vi "basic_serial_write_and_read.vi"(0 "VISA resource name":refnum<visa-resource-name>="COM1", 1 "baud rate":u32=9600, 2 "data bits":u16=8 min=5 max=8 step=1, 3 "parity":u16(ring) items=["None", "Odd", "Even", "Mark", "Space"], 4 "stop bits":u16(ring)=10 items=["1.0"=10, "1.5"=15, "2.0"=20], 7 "flow control":u16(ring) items=["None"=0, "XON/XOFF"=1, "RTS/CTS"=2, "DTR/DSR"=4], 10 "bytes to read":u32=5) -> (9 "read string":string)   [LabVIEW 2017]
doc: "The Basic Serial Read and Write example performs a Serial Port Read, a Serial Port Write, or a combination of these actions. The user selects the actions (read or write) on the front panel. If both are selected, the VI will write the data first, read data, and then close the VISA session that is opened to the port. This VI will wait until the specified number of bytes is received at the port. Only the number of bytes specified will be read.\n\nINSTRUCTIONS:\n1) Select the serial resource and configuration parameters (baud rate, data bits, parity, stop bits, flow control).\n2) Select the operations to be performed. \n3) Connect the serial port to your device. If no device is available, perform a loopback test by doing one of the following. Short pins 2 and 3 on a RS-232 cable or short pin 4 to pin 8 and pin 5 to pin 9 on a RS-485/422 cable. \n4) Run the VI to see the data read. (The \"read string\" will match the \"string to write\" if a loopback test was performed.)\n\nNote: The parameters set for the serial port must match the parameters of the connected instrument or device. In this example, the bytes to read parameter specifies the number of bytes that the serial port reads. If there were more bytes at the port than the number specified in bytes to read, those bytes would not be read. Also, if you specify to read more bytes than the number of bytes actually read, you might receive a timeout error message.\n\nOn the block diagram, the Configure Serial Port VI sets the configuration parameters. The front panel displays the controls used to configure the basic parameters, such as baud rate, data bits, and parity. Constants configure the other parameters the user probably does not need set. After the VISA Configure Serial Port VI opens the VISA session and configures the port, the VI passes the VISA resource name to other VIs that perform operations on that VISA resource. The VISA Write function sends a command to the serial device and the VISA Read function returns data based on the command. The VISA Close function then closes the reference to the serial device. It is important to close the reference; otherwise communication through with that port through protocols other than VISA might not be possible."
uses:
  <vilib>/Instr/_visa.llb/VISA Configure Serial Port (Instr).vi
panel:
  out "x-y":dbl
  out "S2":dbl
  out "S1":dbl
  out "S2":dbl
  out "S1":dbl
  out "output 2":dbl
  out "output 1":dbl
  in  "stop 2":bool
  out "concatenated string":string
  in  "stop":bool
  # "Select the serial resource and the operations (Read, Write, or both) to be performed.  If both are selected, the VI will write the data first, read data and then close the VISA session that is opened to the port.  This VI will wait until the specified number of bytes is received at the port. Only the number of bytes specified will be read."
  # "For additional information select File >> VI Properties >> Documentation"
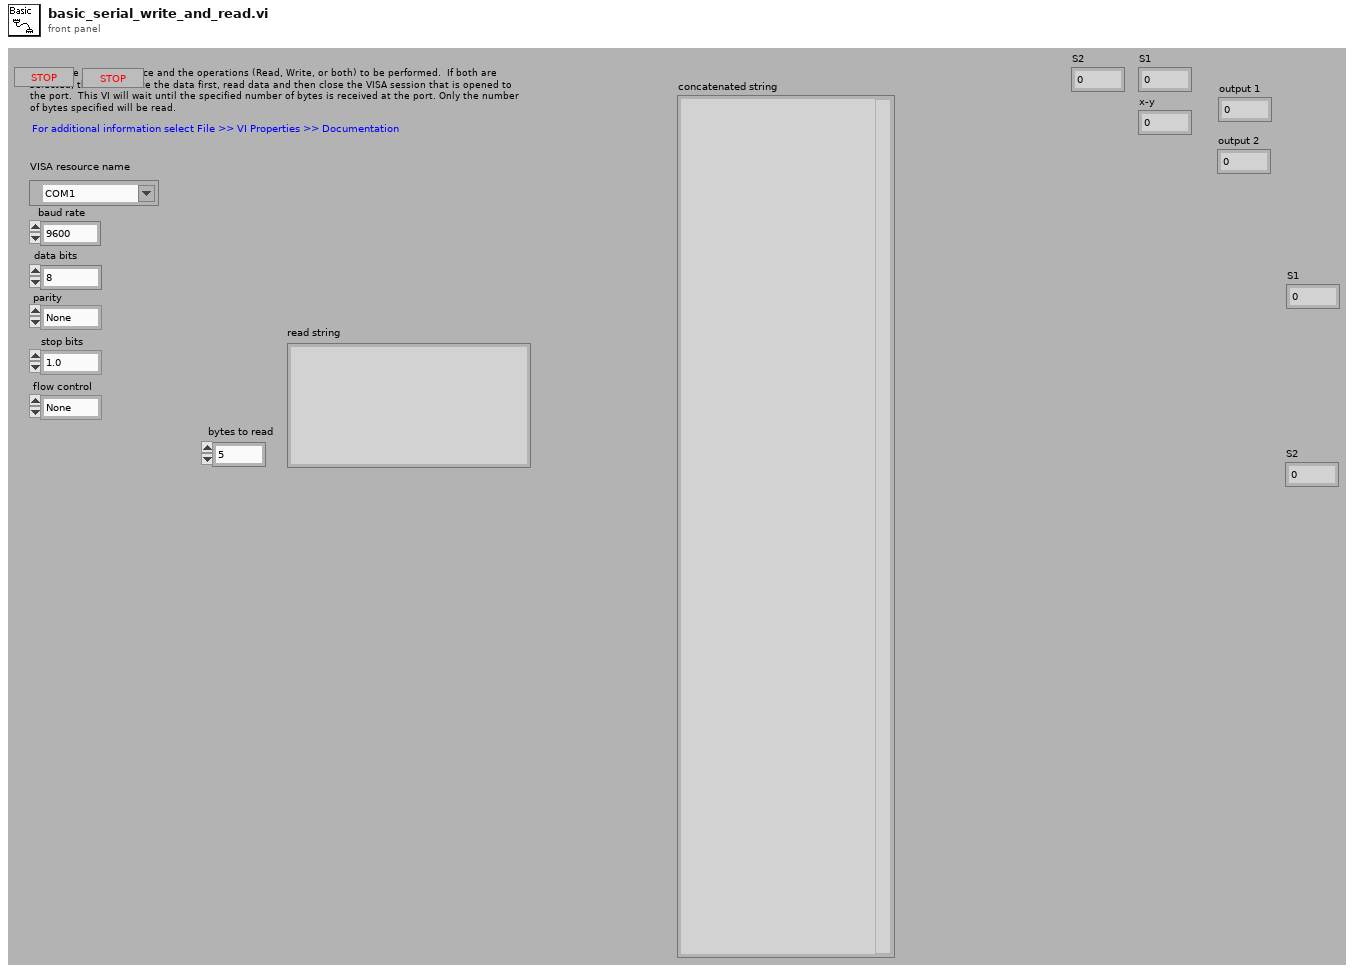
[diagram p1: front panel]
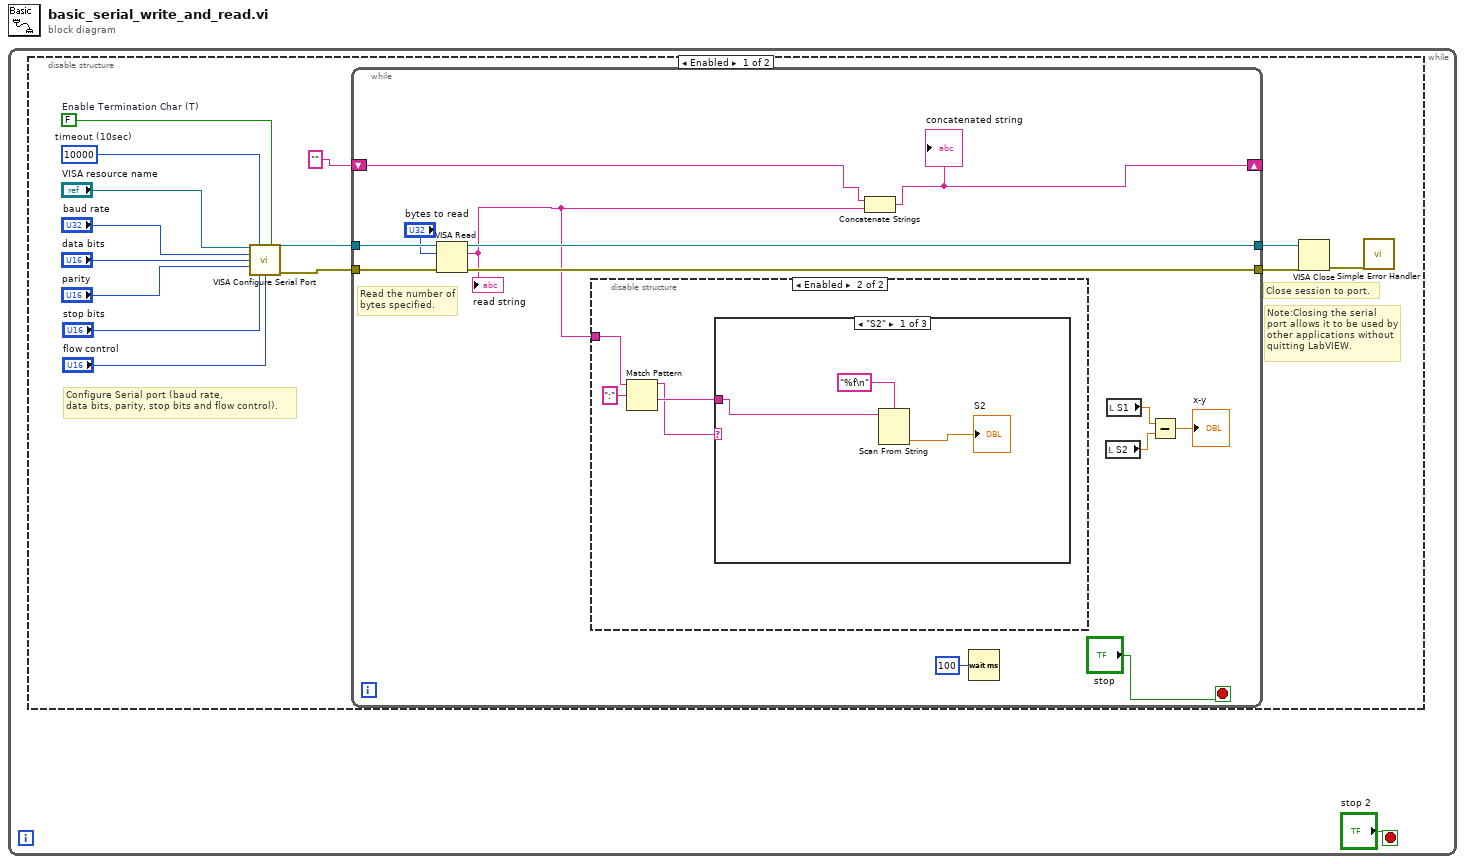
[diagram p0: block diagram]
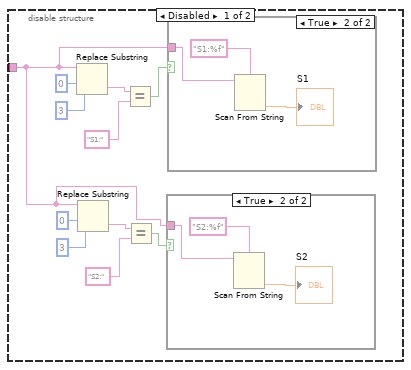
[diagram p2: hidden frame]
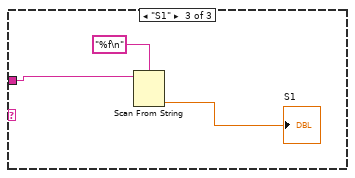
[diagram p6: hidden frame]
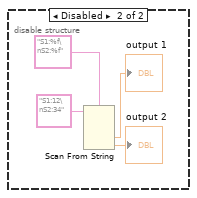
[diagram p7: hidden frame]
diagram:
  n1 = while {
    stop <- "stop 2" stop-if-true
    n2 = disable-structure shown="Enabled" {
      frame Enabled {
        w8 = FALSE  # Enable Termination Char (T)
        w9 = u32 10000  # timeout (10sec)
        # "Note:Closing the serial port allows it to be used by other applications without\nquitting LabVIEW."
        # "Close session to port."
        # "Configure Serial port (baud rate,\ndata bits, parity, stop bits and flow control)."
        n3 = call-poly "VISA Configure Serial Port"("VISA resource name"="VISA resource name", "timeout (10sec)"=w9, "Enable Termination\nChar (T)"=w8, "baud rate (9600)"="baud rate", "data bits (8)"="data bits", "parity (0:none)"="parity", "stop bits (10: 1 bit)"="stop bits", "flow control (0:none)"="flow control") -> ("VISA resource name out"=w11:refnum<visa-resource-name>, "error out"=w12:errorcluster)  [unwired: 6 in]
        n4 = while {
          tunnel: w12 -> [w21]
          tunnel: w11 -> [w22]
          shift-right: [w27] -> _
          shift-left: "" -> [w28]
          tunnel: [w24] -> w3
          tunnel: [w23] -> w2
          stop <- "stop" stop-if-true
          # "Read the number of bytes specified."
          n5 = VISA Read(VISA resource name=w22, byte count="bytes to read", error in (no error)=w21) -> (VISA resource name out=w23:refnum<visa-resource-name>, read buffer=w19:string, error out=w24:errorcluster)  [unwired: 1 out]
          "read string" <- w19
          n6 = disable-structure shown="Enabled" {
            disable-tunnel: w19 -> [w30 w46]
            frame Disabled {
              n7 = Replace Substring(2:3 ("length (len. of substring)"), 3:0 ("offset (0)"), 5:w30) -> (0:w37:string)  [unwired: 1 in, 1 out]
              n8 = Replace Substring(2:3 ("length (len. of substring)"), 3:0 ("offset (0)"), 5:w30) -> (0:w33:string)  [unwired: 1 in, 1 out]
              n9 = Equal?(x=w37, y="S1:") -> (x = y?=w35:bool)
              n10 = Equal?(x=w33, y="S2:") -> (x = y?=w29:bool)
              n11 = case shown="True" w29 {
                tunnel: w30 -> [_ w42]
                frame False {
                }
                frame True {
                  n12 = Scan From String(format string="S2:%f", input string=w42) -> (output 1=→"S2":dbl)  [unwired: 3 in, 3 out]
                }
              }
              n13 = case shown="True" w35 {
                tunnel: w30 -> [_ w45]
                frame False {
                }
                frame True {
                  n14 = Scan From String(format string="S1:%f", input string=w45) -> (output 1=→"S1":dbl)  [unwired: 3 in, 3 out]
                }
              }
            }
            frame Enabled {
              n15 = Match Pattern(string=w46, regular expression=":") -> (before substring=w48:string, after substring=w49:string)  [unwired: 1 in, 2 out]
              n16 = case shown="\"S2\"" w48 {
                tunnel: w49 -> [w50 _ w55]
                frame "S2" {
                  n17 = Scan From String(format string="%f\n", input string=w50) -> (output 1=→"S2":dbl)  [unwired: 3 in, 3 out]
                }
                frame Default {
                }
                frame "S1" {
                  n18 = Scan From String(format string="%f\n", input string=w55) -> (output 1=→"S1":dbl)  [unwired: 3 in, 3 out]
                }
              }
            }
          }
          n19 = Concatenate Strings(w28, w19) -> (w27:string)
          "concatenated string" <- w27
          n20 = Wait (ms)(milliseconds to wait=u32 100) -> ()  [unwired: 1 out]
          n21 = local read "S2"() -> (w17:dbl)
          n22 = local read "S1"() -> (w18:dbl)
          n23 = Subtract(x=w18, y=w17) -> (x-y=→"x-y":dbl)
        }
        n24 = VISA Close(VISA resource name=w2, error in (no error)=w3) -> (error out=w4:errorcluster)
        n25 = call <vilib>:"Simple Error Handler.vi"("error in (no error)"=w4) -> ()  [unwired: 4 in, 5 out]
      }
      frame Disabled {
        n26 = Scan From String(format string="S1:%f\nS2:%f", input string="S1:12\nS2:34") -> (output 1=→"output 1":dbl, output 2=→"output 2":dbl)  [unwired: 4 in, 3 out]
      }
    }
  }
